vi "Core Action.vi"(8 "error in (no error)":errorcluster, 10 "SECS-II Class":refnum<class "SECS-II Class.lvclass">, 11 "23-Equipment Sends Information to Host in":refnum<class "23-Equipment Sends Information to Host.lvclass">) -> (0 "error out":errorcluster, 2 "SECS-II Class Out":refnum<class "SECS-II Class.lvclass">, 3 "23-Equipment Sends Information to Host out":refnum<class "23-Equipment Sends Information to Host.lvclass">)   [LabVIEW 2020, in "SECS Scenarios.lvlib" / "23-Equipment Sends Information to Host.lvclass"]
uses:
  23-Equipment Sends Information to Host.lvclass
  D:/Dropbox/SECS/SECS_GEM v1.1.0/Com/SECS Scenarios/Scenarios Class/Scenarios Class.lvclass
  SECS Communication/SECS-II Class/SECS-II Class.lvclass
  SECS Communication/S10 Message Class/S10F1.ctl
  SECS Communication/S10 Message Class/S10 Message Class.lvclass
  D:/Dropbox/SECS/SECS_GEM v1.1.0/Com/SECS Communication/SECS-II Class/SECS-II Class.lvclass
  23-Equipment Sends Information to Host.lvclass/23-Equipment Sends Information to Host.ctl
  Scenarios Class/Scenarios Class.lvclass/Scenarios Class.ctl
  Scenarios Class/Reply State.ctl
  Scenarios Class/Write Reply State.vi
  Scenarios Class/Read HSMS Class.vi
  SECS Communication/HSMS Class/HSMS Class.lvclass
  Scenarios Class/Scenarios Class.lvclass
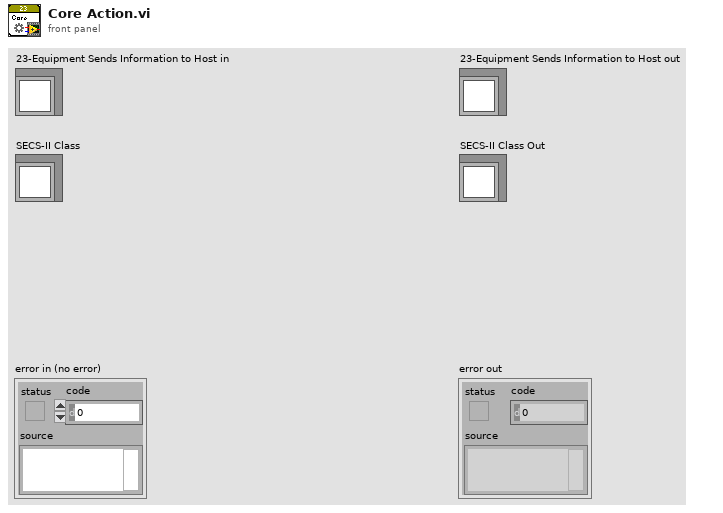
[diagram p1: front panel]
types:
  T1 = typedef "SECS Communication.lvlib/S10 Message Class.lvclass/S10F1.ctl" = cluster{"TID":u8, "TEXT":string}
  T2 = typedef "SECS Scenarios.lvlib/Scenarios Class.lvclass/Reply State.ctl" = enum16{"OK", "Illegal Data", "Unknown Stream", "Unknown Function", "Off-Line", "T3 Timeout", "Inner-Timeout"}
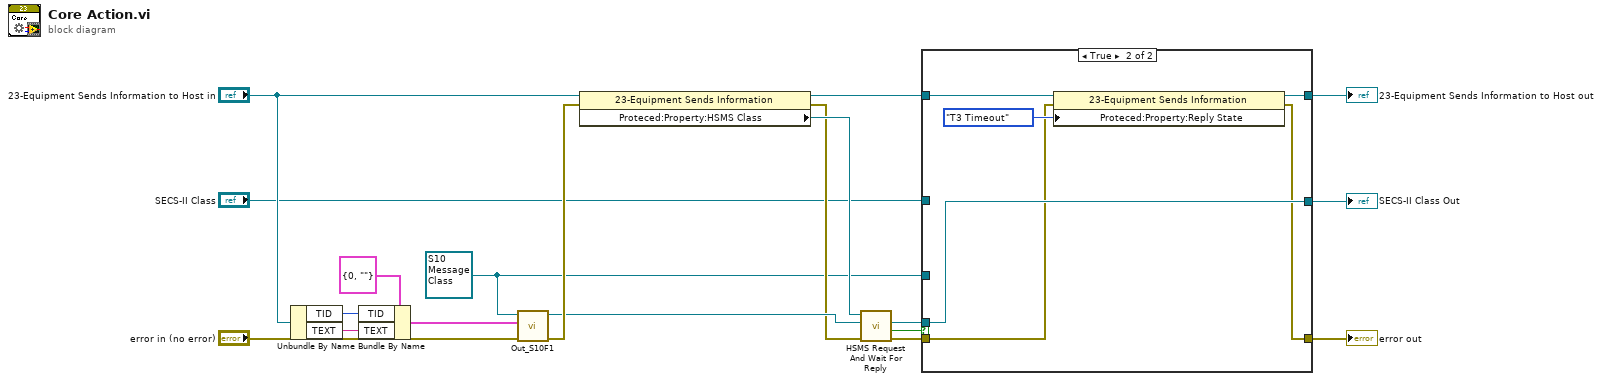
[diagram p0: block diagram]
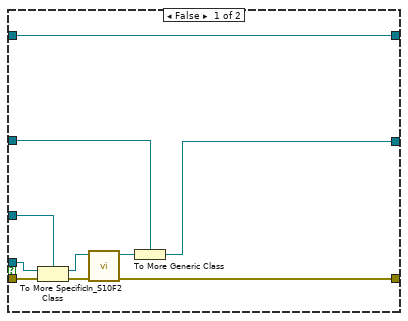
[diagram p2: hidden frame]
diagram:
  w6 = refnum<class "S10 Message Class.lvclass"> refnum ("S10 Message Class in")
  n1 = Unbundle By Name("23-Equipment Sends Information to Host in") -> ("TID"=w18:u8, "TEXT"=w17:string)
  n2 = Bundle By Name(cluster=T1 {"TID"=0, "TEXT"=""} ("S10F1"), "TID"=w18, "TEXT"=w17) -> (w15:T1)
  n3 = call "Out_S10F1.vi"("error in (no error)"="error in (no error)", "S10F1"=w15, "S10 Message Class in"=w6) -> ("error out"=w13:errorcluster, "S10 Message Class out"=w12:refnum<class "S10 Message Class.lvclass">)  [unwired: 7 in]
  n4 = property class="23-Equipment Sends Information "(reference="23-Equipment Sends Information to Host in", error in=w13) -> (reference out=w4:refnum<class "23-Equipment Sends Information to Host.lvclass">, error out=w10:errorcluster, "Proteced:Property:HSMS Class"=w11:refnum<class "HSMS Class.lvclass">)
  n5 = call "HSMS Request And Wait For Reply.vi"("error in (no error)"=w10, "SECS-II Class In"=w12, "HSMS Class in"=w11) -> ("error out"=w9:errorcluster, "Timeout?"=w8:bool, "SECS-II Class Out"=w7:refnum<class "SECS-II Class.lvclass">)  [unwired: 5 in, 1 out]
  n6 = case shown="True" w8 {
    tunnel: w9 -> [w29 w31]
    tunnel: w7 -> [w28 w35]
    tunnel: w6 -> [w27 _]
    tunnel: [w24 w30] -> w5
    tunnel: w4 -> [w23 w34]
    tunnel: [w23 w33] -> w3
    tunnel: "SECS-II Class" -> [w21 _]
    tunnel: [w20 w35] -> w1
    frame False {
      n7 = To More Specific Class(target class=w27, reference=w28, error in=w29) -> (specific class reference=w25:refnum<class "S10 Message Class.lvclass">, error out=w26:errorcluster)
      n8 = call "In_S10F2.vi"("error in (no error)"=w26, "S10 Message Class in"=w25) -> ("error out"=w24:errorcluster, "S10 Message Class out"=w22:refnum<class "S10 Message Class.lvclass">)  [unwired: 6 in, 2 out]
      n9 = To More Generic Class(target class=w21, reference=w22) -> (generic class reference=w20:refnum<class "SECS-II Class.lvclass">)
    }
    frame True {
      n10 = property class="23-Equipment Sends Information "(reference=w34, error in=w31, "Proteced:Property:Reply State"=Reply_State."T3 Timeout" ("Reply State")) -> (reference out=w33:refnum<class "23-Equipment Sends Information to Host.lvclass">, error out=w30:errorcluster)
    }
  }
  "error out" <- w5
  "23-Equipment Sends Information to Host out" <- w3
  "SECS-II Class Out" <- w1
